vi "TOOLweb POLL.vi"(4 "error in (no error)":errorcluster caption="Fehler (Eingang, kein Fehler)", 5 "IP-Adresse (localhost)":string="127.0.0.1", 7 "EVID-Nummer":i32=1) -> (0 "error out":errorcluster caption="Fehler (Ausgang)", 3 "Wert-String":string)   [LabVIEW 2020, in "FT-IR.lvlib" / "TOOLweb Interface.lvlib"]
doc: "Holt mit einer HTTP-POST-Anforderung gemäß TOOLweb-Protokoll den Wert einer einzigen Variablen (EVID-Nummer) als \"Wert-String\" vom MKS MultiGas 2030 Analyzer. \n\nFalls der TOOLWeb-Server nicht auf demselben Rechner arbeitet, kann mit \"IP-Adresse\" eine beliebiger Host adressiert werden. Ein unverbundener Eingang spricht den lokalen Host an."
uses:
  TOOLweb Interface.lvlib
  TOOLweb Interface Hilfs-VIs.lvlib
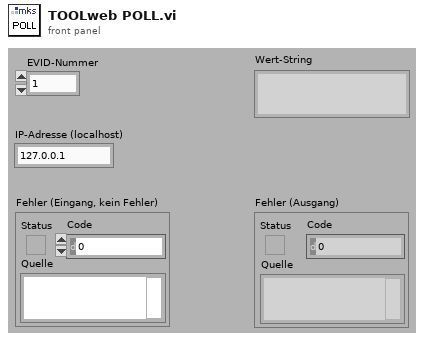
[diagram p1: front panel]
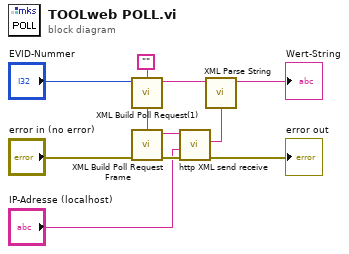
[diagram p0: block diagram]
diagram:
  n1 = call "XML Build Poll Request(1).vi"("XML-Message alt"="", "EVID-Nummer"="EVID-Nummer") -> ("Attribut Name"=w8:string, "XML-Message neu"=w2:string)  [unwired: 6 out]
  n2 = call "XML Build Poll Request Frame.vi"("XML-Message"=w2, "error in (no error)"="error in (no error)") -> ("XML-Message fertig"=w7:string, "error out"=w10:errorcluster)  [unwired: 1 in, 5 out]
  n3 = call "http XML send receive.vi"("error in (no error)"=w10, "IP-Adresse (localhost)"="IP-Adresse (localhost)", "XML Request"=w7) -> ("error out"=→"error out":errorcluster, "Response Body (XML)"=w1:string)  [unwired: 3 out]
  n4 = call "XML Parse String.vi"("Attribut Name"=w8, "XML Response"=w1) -> ("Wert-String"=→"Wert-String":string)  [unwired: 7 out]
